vi "Process Name.vi"() -> (3 "process name":string)   [LabVIEW 2021, in "TemplateProcess.lvlib"]
uses:
  TemplateProcess.lvlib
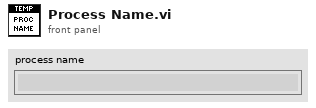
[diagram p1: front panel]
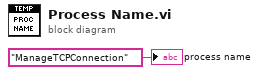
[diagram p0: block diagram]
diagram:
  "process name" <- "ManageTCPConnection" ("ProcessName")
